vi "Read Time.vi"(8 "error in (no error)":errorcluster, 11 "Shutter in":refnum<class "Shutter.lvclass">) -> (0 "error out":errorcluster, 2 "Time Stamp":timestamp, 3 "Shutter out":refnum<class "Shutter.lvclass">)   [LabVIEW 2016, in "Shutter.lvclass"]
uses:
  Shutter.lvclass
  Shutter.lvclass/Shutter.ctl
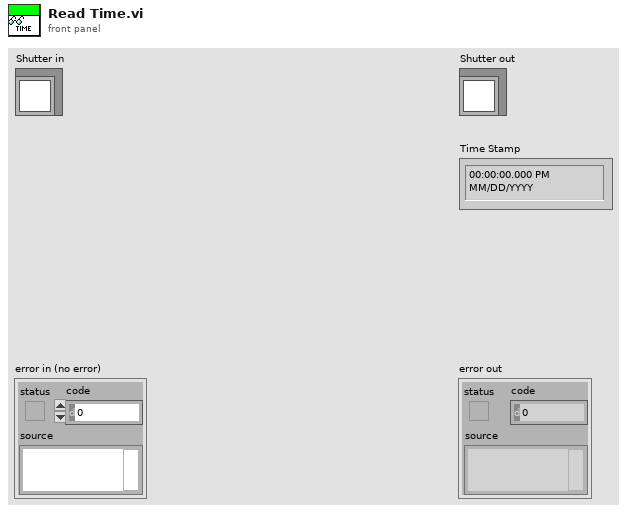
[diagram p1: front panel]
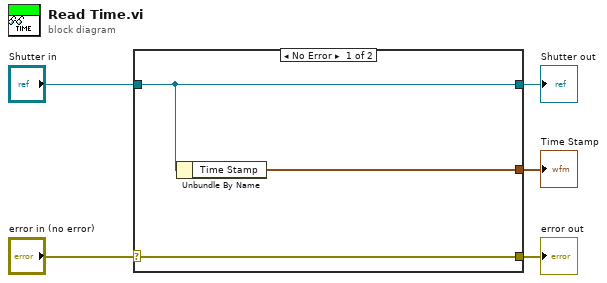
[diagram p0: block diagram]
diagram:
  n1 = case shown="No Error" "error in (no error)" {
    selector: "error in (no error)" -> [w8 w9]
    tunnel: [w8 w9] -> w4
    tunnel: [w7 w10] -> w2
    tunnel: "Shutter in" -> [w7 w10]
    tunnel: [w6 _] -> w1
    frame No Error {
      n2 = Unbundle By Name(w7) -> ("Time Stamp"=w6:timestamp)
    }
    frame Error {
    }
  }
  "error out" <- w4
  "Shutter out" <- w2
  "Time Stamp" <- w1
